vi "TeleopAutoBalance.vi"(10 "Match Info":T1={"Autonomous Elapsed Seconds"=0.0, "TeleOp Elapsed Seconds"=0.0, "Disabled Elapsed Seconds"=0.0, "Visited Autonomous"=FALSE, "Visited TeleOp"=FALSE, "Visited Disabled"=FALSE, "Autonomous Settings"={"Autonomous Style"=enum."Independent", "VI Refnum"=refnum}}, 11 "Call Context":T2) -> ()   [LabVIEW 2016, in "navX Library.lvlib"]
doc: "This VI is called for each TeleOp packet received from the DS where the robot is not disabled. It is often used to read from the joysticks and update I/O or to update setpoints for timed control loops. It should complete and return within 20 milliseconds or it may miss DS packets."
uses:
  navX Library.lvlib
  <vilib>/Rock Robotics/WPI/DriverStation/WPI_DriverStationDerivedRobotMode.ctl
  <vilib>/Rock Robotics/WPI/DriverStation/WPI_DriverStationMatch Info.ctl
  _TypeDefs/FRIC_navX_DeviceNumbersTypeDef.ctl
  <vilib>/Rock Robotics/WPI/Utilities/WPI_GetSetVariantRefNum.vi
  <vilib>/Rock Robotics/Network Tables/SD Write Boolean Array.vi
  <vilib>/Rock Robotics/Network Tables/SD Write Numeric Array.vi
  <vilib>/Rock Robotics/Network Tables/SD Read Boolean.vi
  <vilib>/Rock Robotics/Network Tables/SD Read Number.vi
  <vilib>/Rock Robotics/WPI/RobotDrive/WPI_RobotDriveMecanumDrive_Cartesian.vi
panel:
  out "Sample Slider 0":dbl(slide) scale=0.0..5.0
  out "Sample Boolean 1":bool
  out "Sample Boolean 0":bool
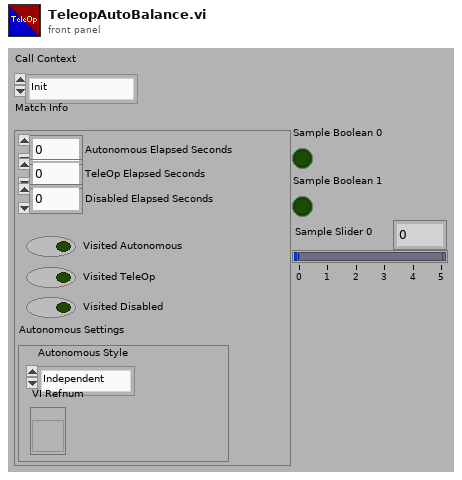
[diagram p1: front panel]
types:
  T1 = typedef "WPI_DriverStationMatch Info.ctl" = cluster{"Autonomous Elapsed Seconds":dbl, "TeleOp Elapsed Seconds":dbl, "Disabled Elapsed Seconds":dbl, "Visited Autonomous":bool, "Visited TeleOp":bool, "Visited Disabled":bool, "Autonomous Settings":cluster{"Autonomous Style":enum16{"Iterative", "Independent"}, "VI Refnum":refnum<vi>}}
  T2 = typedef "WPI_DriverStationDerivedRobotMode.ctl" = enum16{"Init", "Execute", "Stop"}
  T3 = typedef "navX Library.lvlib/FRIC_navX_DeviceNumbersTypeDef.ctl" = enum16{"Dev0", "Dev1", "Dev2", "Dev3"}
  T4 = typedef "WPI_JoystickDevRef.ctl" = cluster{"Device":T5}
  T5 = typedef "WPI_JoystickDeviceEnum.ctl" = enum16{"USB 0", "USB 1", "USB 2", "USB 3", "USB 4", "USB 5"}
  T6 = typedef "WPI_RobotDriveDevRef.ctl" = cluster{"DevStatus":errorcluster, "Motors[]":T7[], "Square Inputs":bool, "Max Output":dbl}
  T7 = typedef "WPI_MotorControlDeviceRef.ctl" = cluster{"DeviceStatus":errorcluster, "Type":T8, "PWM":cluster{"PWM Channel":T9, "DeadBand":T10}, "CAN":cluster{"Device Number":u8, "SetOutput VI Ref":variant, "GetOutput VI Ref":variant, "Enable VI Ref":variant, "Disable VI Ref":variant, "Data":variant}, "Invert":bool}
  T8 = typedef "WPI_MotorControlType.ctl" = enum16{"PWM", "CAN"}
  T9 = typedef "FPGA_DIOPWMChannel.ctl" = enum8{"PWM 0", "PWM 1", "PWM 2", "PWM 3", "PWM 4", "PWM 5", "PWM 6", "PWM 7", "PWM 8", "PWM 9", "PWM MXP 0", "PWM MXP 1", "PWM MXP 2", "PWM MXP 3", "PWM MXP 4", "PWM MXP 5", "PWM MXP 6", "PWM MXP 7", "PWM MXP 8", "PWM MXP 9", "Invalid"}
  T10 = typedef "WPI_PWMDeadband.ctl" = cluster{"Name":string, "maxPositivePwm":i32, "minPositivePwm":i32, "centerPwm":i32, "maxNegativePwm":i32, "minNegativePwm":i32, "angularRange":u16}
  T11 = cluster{"Yaw":dbl, "Roll":dbl, "Pitch":dbl, "Heading":dbl, "Fused Heading":dbl}
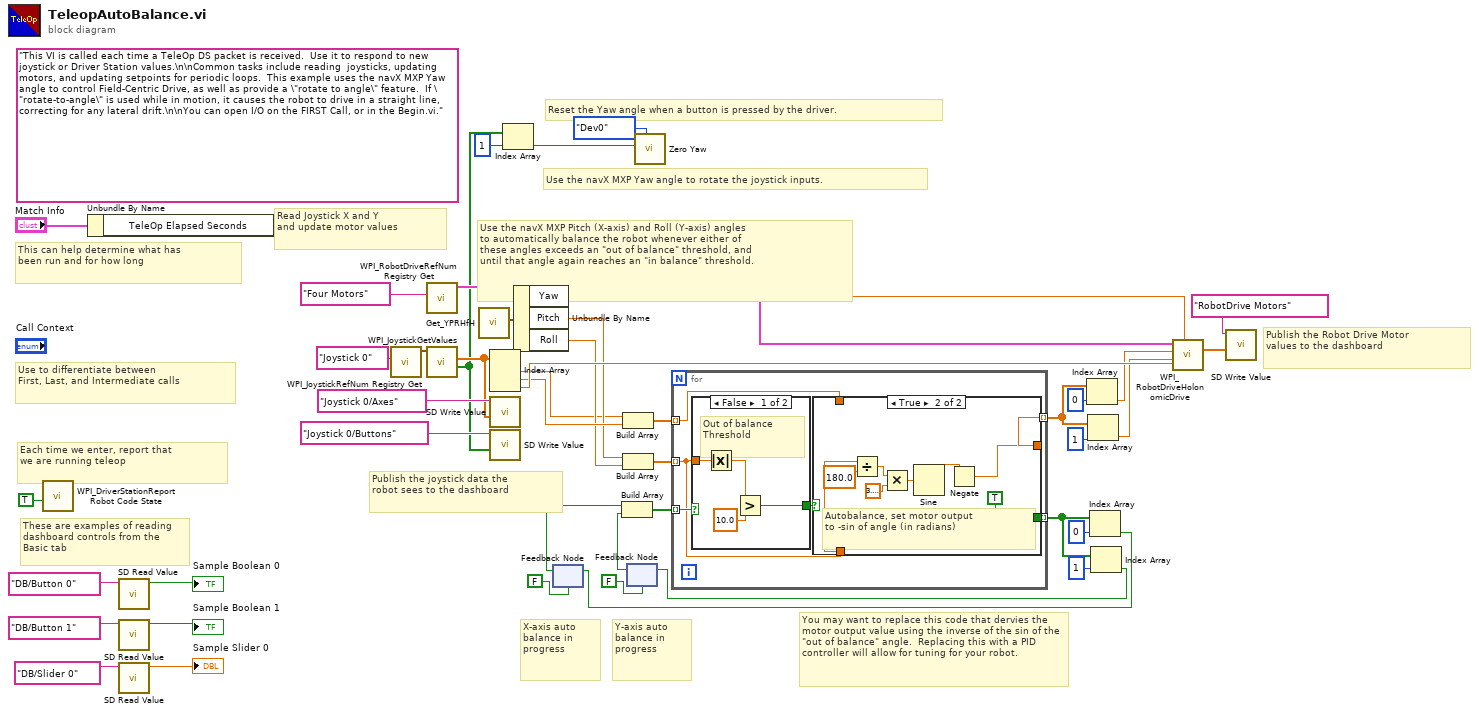
[diagram p0: block diagram]
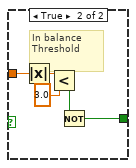
[diagram p2: hidden frame]
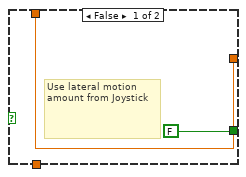
[diagram p3: hidden frame]
diagram:
  (unwired) "This VI is called each time a TeleOp DS packet is received.  Use it to respond to new joystick or Driver Station values.\n\nCommon tasks include reading  joysticks, updating motors, and updating setpoints for periodic loops.  This example uses the navX MXP Yaw angle to control Field-Centric Drive, as well as provide a \"rotate to angle\" feature.  If \"rotate-to-angle\" is used while in motion, it causes the robot to drive in a straight line, correcting for any lateral drift.\n\nYou can open I/O on the FIRST Call, or in the Begin.vi."
  # "Reset the Yaw angle when a button is pressed by the driver."
  # "You may want to replace this code that dervies the motor output value using the inverse of the sin of the \"out of balance\" angle.  Replacing this with a PID controller will allow for tuning for your robot."
  # "Y-axis auto\nbalance in \nprogress"
  # "X-axis auto\nbalance in \nprogress"
  # "Use the navX MXP Pitch (X-axis) and Roll (Y-axis) angles\nto automatically balance the robot whenever either of \nthese angles exceeds an \"out of balance\" threshold, and\nuntil that angle again reaches an \"in balance\" threshold."
  # "Use the navX MXP Yaw angle to rotate the joystick inputs."
  # "These are examples of reading dashboard controls from the Basic tab"
  # "Publish the Robot Drive Motor\nvalues to the dashboard"
  # "Publish the joystick data the\nrobot sees to the dashboard"
  # "Each time we enter, report that\nwe are running teleop"
  # "Use to differentiate between\nFirst, Last, and Intermediate calls"
  # "This can help determine what has\nbeen run and for how long"
  # "Read Joystick X and Y \nand update motor values"
  n1 = call <vilib>:"WPI_DriverStationReport Robot Code State.vi"("TeleOp"=TRUE ("Autonomous")) -> ()  [unwired: 10 in, 1 out]
  n2 = Unbundle By Name("Match Info") -> ()  [unwired: 1 out]
  n3 = call-poly <vilib>:"SD Read Value.vi"("Name"="DB/Button 0" ("refnum name")) -> ("Boolean"=→"Sample Boolean 0":bool)  [unwired: 8 in, 2 out]
  n4 = call-poly <vilib>:"SD Read Value.vi"("Name"="DB/Button 1" ("refnum name")) -> ("Boolean"=→"Sample Boolean 1":bool)  [unwired: 8 in, 2 out]
  n5 = call-poly <vilib>:"SD Read Value.vi"("Name"="DB/Slider 0" ("refnum name")) -> ("Numeric"=→"Sample Slider 0":dbl)  [unwired: 8 in, 2 out]
  n6 = call <vilib>:"WPI_JoystickRefNum Registry Get.vi"("refnum name"="Joystick 0") -> ("JoystickDevRef"=w41:T4)  [unwired: 1 in, 9 out]
  n7 = call <vilib>:"WPI_RobotDriveRefNum Registry Get.vi"("refnum name"="Four Motors") -> ("RobotDriveDevRef"=w43:T6)  [unwired: 1 in, 9 out]
  n8 = call <vilib>:"WPI_JoystickGetValues.vi"("JoystickDevRef"=w41) -> ("Buttons"=w26:bool[], "Axes"=w29:dbl[])  [unwired: 6 in, 3 out]
  n9 = call "Get_YPRHfH.vi"() -> ("YRPHfH"=w3:T11)  [unwired: 11 in]
  n10 = Index Array(array=w29) -> (element #1=w4:dbl, element #2=w8:dbl, element #3=w25:dbl)  [unwired: 3 in]
  n11 = call-poly <vilib>:"SD Write Value.vi"("Numeric Array"=w29, "Name"="Joystick 0/Axes") -> ()  [unwired: 8 in, 2 out]
  n12 = call-poly <vilib>:"SD Write Value.vi"("Boolean Array"=w26, "Name"="Joystick 0/Buttons") -> ()  [unwired: 8 in, 2 out]
  n13 = Index Array(array=w26, index=1) -> (element=w2:bool)
  n14 = Unbundle By Name(w3) -> ("Yaw"=w27:dbl, "Pitch"=w7:dbl, "Roll"=w6:dbl)
  n15 = feedback #1(FALSE) -> (w22:bool)
  n16 = Build Array(w4, w8) -> (w19:dbl[])
  n17 = Build Array(w7, w6) -> (w5:dbl[])
  n18 = feedback #2(FALSE) -> (w21:bool)
  n19 = Build Array(w22, w21) -> (w20:bool[])
  n20 = call "Zero Yaw.vi"("Device Number"=FRIC_navX_DeviceNumbersTypeDef."Dev0", "Zero"=w2) -> ()  [unwired: 10 in]
  n21 = for {
    tunnel: w20 -> [w50] mode=indexing
    tunnel: w19 -> [w46] mode=indexing
    tunnel: [w49] -> w18 mode=indexing
    tunnel: [w48] -> w11 mode=indexing
    tunnel: w5 -> [w47] mode=indexing
    n22 = case shown="False" w50 {
      tunnel: w47 -> [w55 w58]
      tunnel: [w52 w57] -> w51
      frame False {
        # "Out of balance\nThreshold"
        n23 = Absolute Value(x=w55) -> (abs(x)=w54:dbl)
        n24 = Greater?(x=w54, y=10.0) -> (0:w52:bool)
      }
      frame True {
        # "In balance\nThreshold"
        n25 = Absolute Value(x=w58) -> (abs(x)=w59:dbl)
        n26 = Less?(x=w59, y=3.0) -> (x < y?=w56:bool)
        n27 = Not(x=w56) -> (.not. x?=w57:bool)
      }
    }
    n28 = case shown="True" w51 {
      tunnel: w47 -> [_ w69]
      tunnel: [w61 w63] -> w48
      tunnel: [FALSE TRUE] -> w49
      tunnel: w46 -> [w61 _]
      frame False {
        # "Use lateral motion amount from Joystick"
      }
      frame True {
        # "Autobalance, set motor output \nto -sin of angle (in radians)"
        n29 = Divide(x=w69, y=180.0) -> (x/y=w67:dbl)
        n30 = Multiply(x=w67, y=3.141592653589793) -> (x*y=w65:dbl)
        n31 = Sine(x=w65) -> (sin(x)=w64:dbl)
        n32 = Negate(x=w64) -> (-x=w63:dbl)
      }
    }
  }
  n33 = Index Array(array=w11, index=0) -> (element=w10:dbl)
  n34 = Index Array(array=w11, index=1) -> (element=w9:dbl)
  n35 = Index Array(array=w18, index=0) -> (element=w15:bool)
  n36 = feedback-in #1(w15) -> ()
  n37 = Index Array(array=w18, index=1) -> (element=w14:bool)
  n38 = feedback-in #2(w14) -> ()
  n39 = call-poly <vilib>:"WPI_RobotDriveHolonomicDrive.vi"("Rotation"=w25, "Gyro Angle"=w27, "Y"=w9, "X"=w10, "RobotDriveDevRef"=w43) -> ("Motor Values"=w30:dbl[])  [unwired: 4 in, 2 out]
  n40 = call-poly <vilib>:"SD Write Value.vi"("Numeric Array"=w30, "Name"="RobotDrive Motors") -> ()  [unwired: 8 in, 2 out]
